vi "Execute.vi"(8 "error in (no error)":errorcluster, 11 "Function Generator in":refnum<class "Function Generator.lvclass">) -> (0 "error out":errorcluster, 2 "Data":dbl[](array[numeric]), 3 "Function Generator out":refnum<class "Function Generator.lvclass">)   [LabVIEW 2021, in "Function Generator.lvclass"]
uses:
  Function Generator.lvclass
  Function Generator.lvclass/Function Generator.ctl
  <vilib>/measure/NI_MABase.lvlib
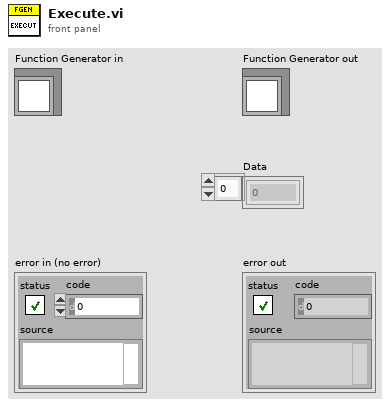
[diagram p1: front panel]
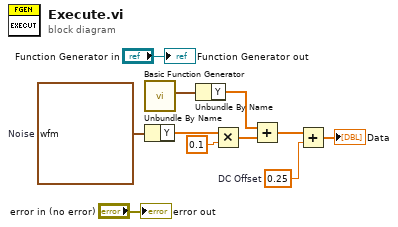
[diagram p0: block diagram]
diagram:
  w4 = 0.25  # DC Offset
  w5 = waveform(dbl) {"t0"=timestamp(0 s since 1904-01-01), "dt"=0.001, "Y"=array[1000 elements]}  # Noise
  n1 = call <vilib>:"Basic Function Generator.vi"() -> ("signal out"=w10:waveform(dbl))  [unwired: 9 in, 2 out]
  n2 = Unbundle By Name(w5) -> ("Y"=w7:dbl[])
  n3 = Unbundle By Name(w10) -> ("Y"=w9:dbl[])
  n4 = Multiply(x=w7, y=0.1) -> (x*y=w3:dbl[])
  n5 = Add(x=w9, y=w3) -> (x+y=w8:dbl[])
  n6 = Add(x=w8, y=w4) -> (x+y=→"Data":dbl[])
  "error out" <- "error in (no error)"
  "Function Generator out" <- "Function Generator in"
